vi "TURBOset.vi"(1 "SV":dbl format="%.1f", 2 "Device number":i8=1, 3 "VISA resource name":refnum<visa-resource-name>) -> (0 "error out":errorcluster)   [LabVIEW 2014]
uses:
  <vilib>/Instr/_visa.llb/VISA Configure Serial Port (Instr).vi
panel:
  out "Data from ATEC302":string
  out "CRC data for ATEC302":string
  out "Upper CRC Byte":u32 format="%x"
  out "Lower CRC Byte":u32 format="%x"
  out "CRC =":u16 format="%x"
  out "Data without CRC":string
  out "DN HEX":string
  out "SV HEX":string
  # "Set temperature"
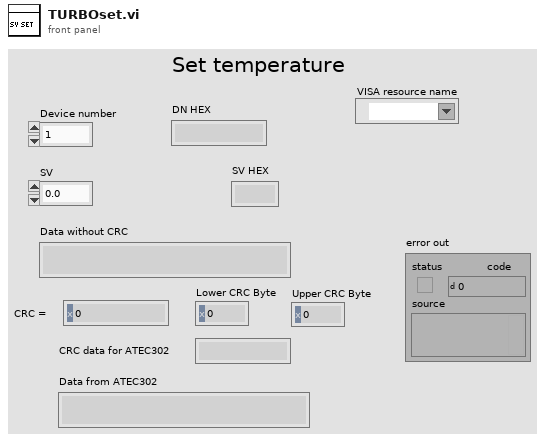
[diagram p1: front panel]
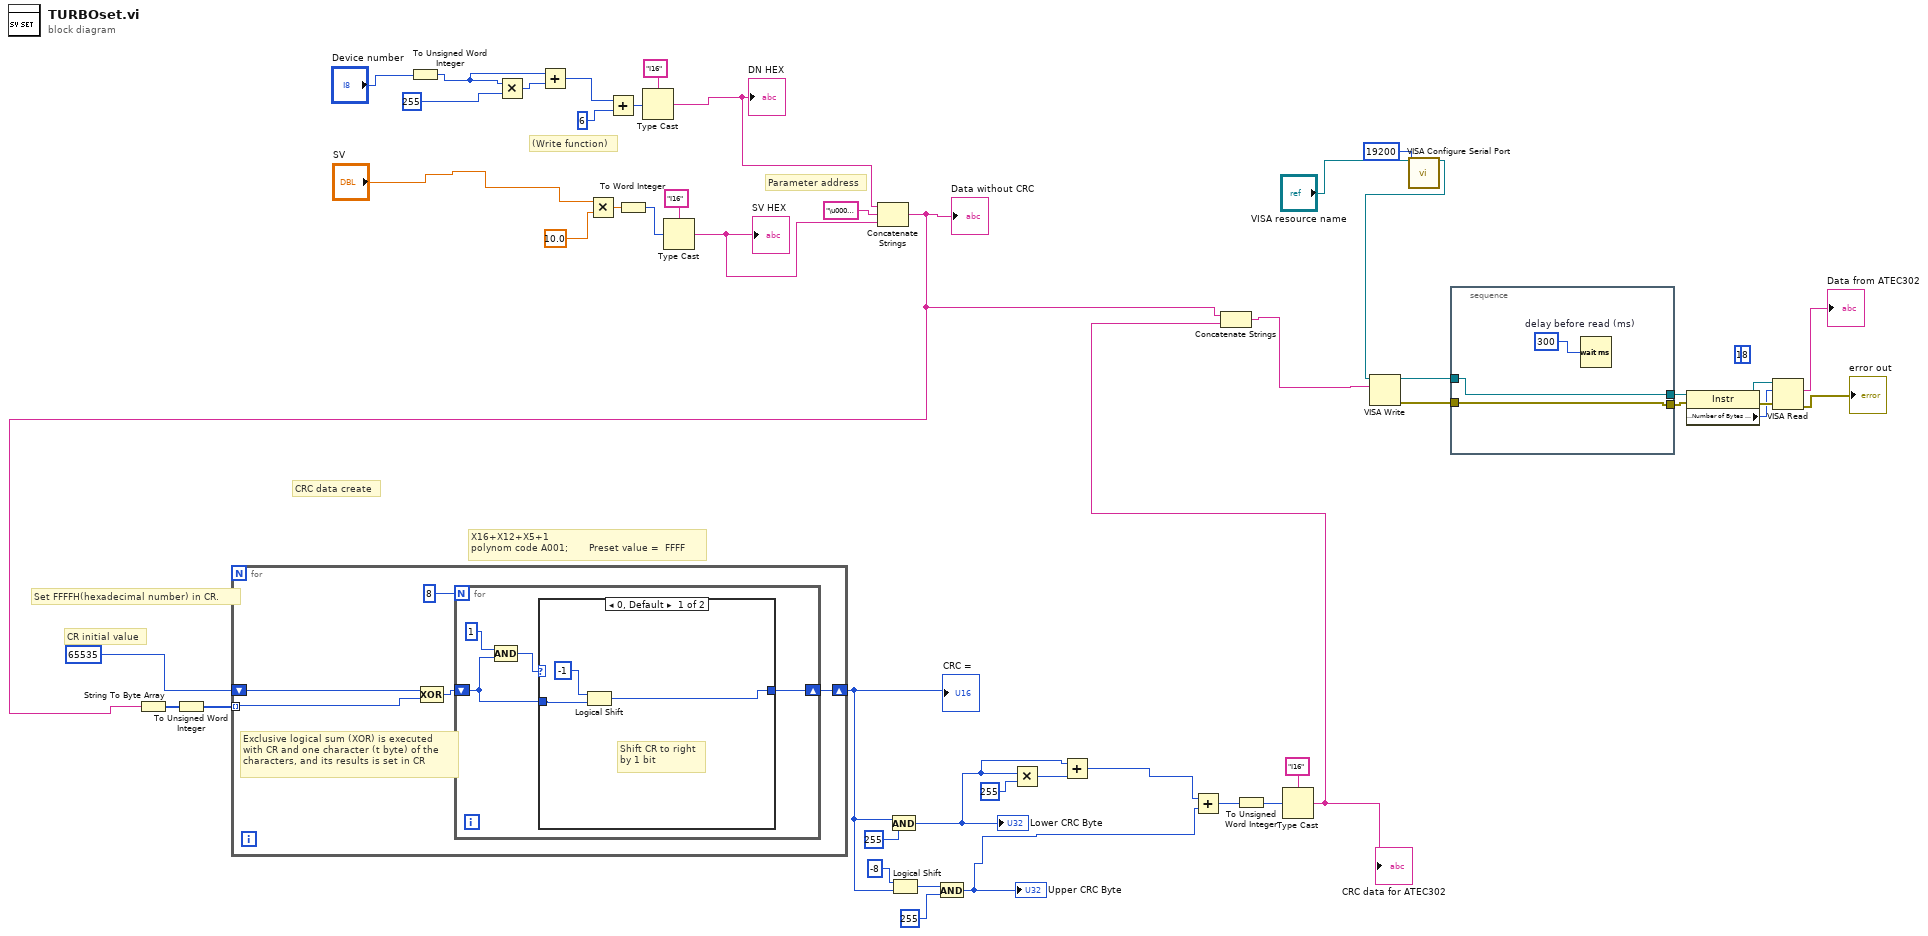
[diagram p0: block diagram]
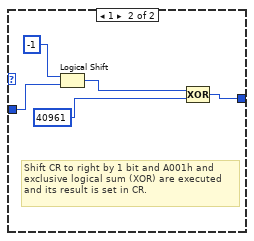
[diagram p2: hidden frame]
diagram:
  (unwired) u16 16 ("y")
  (unwired) u16 8 ("y")
  # "Parameter address"
  # "CRC data create"
  # "Set FFFFH(hexadecimal number) in CR."
  # "CR initial value"
  # "X16+X12+X5+1\npolynom code A001;       Preset value =  FFFF"
  # "(Write function)"
  n1 = To Unsigned Word Integer(number="Device number") -> (unsigned 16bit integer=w36:u16)
  n2 = Multiply(x=w36, y=u16 255) -> (x*y=w38:u16)
  n3 = Add(x=w36, y=w38) -> (x+y=w37:u16)
  n4 = Multiply(x="SV", y=10.0) -> (x*y=w46:dbl)
  n5 = Add(x=w37, y=u16 6) -> (x+y=w39:u16)
  n6 = To Word Integer(number=w46) -> (16bit integer=w45:i16)
  n7 = Type Cast(type="I16", x=w39) -> (*(type *) &x=w35:string)
  "DN HEX" <- w35
  n8 = Type Cast(type="I16", x=w45) -> (*(type *) &x=w34:string)
  "SV HEX" <- w34
  n9 = Concatenate Strings(w35, "\u0000\u0000", w34) -> (w18:string)
  "Data without CRC" <- w18
  n10 = String To Byte Array(string=w18) -> (unsigned byte array=w32:u8[])
  n11 = To Unsigned Word Integer(number=w32) -> (unsigned 16bit integer=w31:u16[])
  n12 = for {
    shift-right: [w49] -> w27
    shift-left: u16 65535 -> [w50]
    tunnel: w31 -> [w48] mode=indexing
    # "Exclusive logical sum (XOR) is executed\nwith CR and one character (t byte) of the\ncharacters, and its results is set in CR"
    n13 = Compound Arithmetic op=XOR(w50, w48) -> (w51:u32)
    n14 = for {
      N: 8 -> [_]
      shift-right: [w55] -> w49
      shift-left: w51 -> [w54]
      n15 = Compound Arithmetic op=AND(u16 1, w54) -> (w53:u32)
      n16 = case shown="0, Default" w53 {
        tunnel: [w58 w63] -> w55
        tunnel: w54 -> [w57 w60]
        frame 0, Default {
          # "Shift CR to right\nby 1 bit"
          n17 = Logical Shift(y=i16 -1, x=w57) -> (x << y=w58:u32)
        }
        frame 1 {
          # "Shift CR to right by 1 bit and A001h and\nexclusive logical sum (XOR) are executed\nand its result is set in CR."
          n18 = Logical Shift(y=i16 -1, x=w60) -> (x << y=w62:u32)
          n19 = Compound Arithmetic op=XOR(w62, u32 40961) -> (w63:u32)
        }
      }
    }
  }
  "CRC =" <- w27
  n20 = And(x=w27, y=u16 255) -> (x .and. y?=w21:u32)
  "Lower CRC Byte" <- w21
  n21 = Logical Shift(y=i16 -8, x=w27) -> (x << y=w28:u32)
  n22 = And(x=w28, y=u16 255) -> (x .and. y?=w24:u32)
  "Upper CRC Byte" <- w24
  n23 = Multiply(x=w21, y=u16 255) -> (x*y=w22:u32)
  n24 = Add(x=w21, y=w22) -> (x+y=w23:u32)
  n25 = Add(x=w23, y=w24) -> (x+y=w16:u32)
  n26 = To Unsigned Word Integer(number=w16) -> (unsigned 16bit integer=w19:u16)
  n27 = Type Cast(type="I16", x=w19) -> (*(type *) &x=w17:string)
  "CRC data for ATEC302" <- w17
  n28 = Concatenate Strings(w18, w17) -> (w15:string)
  n29 = call-poly "VISA Configure Serial Port"("VISA resource name"="VISA resource name", "baud rate (9600)"=u32 19200) -> ("VISA resource name out"=w2:refnum<visa-resource-name>)  [unwired: 12 in, 1 out]
  n30 = VISA Write(VISA resource name=w2, write buffer=w15) -> (VISA resource name out=w10:refnum<visa-resource-name>, error out=w7:errorcluster)  [unwired: 1 in, 1 out]
  n31 = stacked-sequence {
    tunnel: w10 -> [w66]
    tunnel: [w66] -> w9
    tunnel: w7 -> [w65]
    tunnel: [w65] -> w6
    frame #0 {
      w67 = u32 300  # delay before read (ms)
      n32 = Wait (ms)(milliseconds to wait=w67) -> ()  [unwired: 1 out]
    }
  }
  n33 = property class="Instr"(reference=w9, error in=w6) -> (reference out=w8:refnum<visa-resource-name>, error out=w12:errorcluster, "Serial Settings:Number of Bytes at Serial Port"=w11:u32)
  n34 = VISA Read(VISA resource name=w8, byte count=w11, error in (no error)=w12) -> (read buffer=→"Data from ATEC302":string, error out=→"error out":errorcluster)  [unwired: 2 out]
